vi "NI VeriStand - Close Percent Complete Notification.vi"(8 "error in (no error)":errorcluster, 11 "PercentComplete Refs":T1) -> (0 "error out":errorcluster)   [LabVIEW 2020, in "NI_VS MacroPlayerAPI.lvlib"]
doc: "Closes an open reference to messages the Macro Player sends that indicate the percentage of the macro file that has played back. Use the Open Percent Complete Notification VI to open the reference this VI closes."
uses:
  <vilib>/NI VeriStand/Execution/MacroPlayer/NI_VS MacroPlayerAPI.lvlib
  <vilib>/NI VeriStand/Execution/MacroPlayer/PercentComplete Refs.ctl
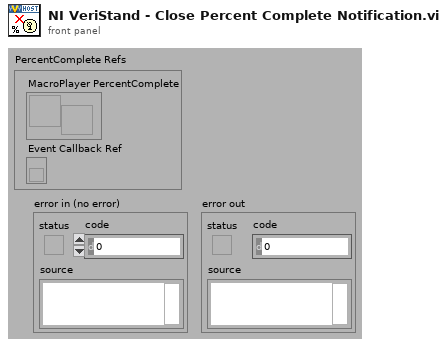
[diagram p1: front panel]
types:
  T1 = typedef "NI_VS MacroPlayerAPI.lvlib/PercentComplete Refs.ctl" = cluster{"MacroPlayer PercentComplete":refnum<user-event>, "Event Callback Ref":refnum<k27>}
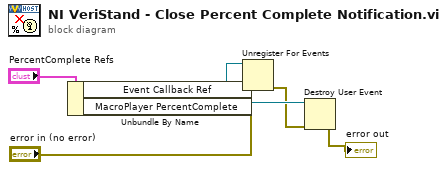
[diagram p0: block diagram]
diagram:
  n1 = Unbundle By Name("PercentComplete Refs") -> ("Event Callback Ref"=w5:refnum<k27>, "MacroPlayer PercentComplete"=w4:refnum<user-event>)
  n2 = Unregister For Events(event registration refnum=w5, error in="error in (no error)") -> (error out=w3:errorcluster)
  n3 = Destroy User Event(user event=w4, error in=w3) -> (error out=→"error out":errorcluster)
